vi "afslag_aan_het_kruispunt (SubVI).vi"(10 "OK Button":bool, 11 "afslag: rechtdoor: d,linksaf: l,rechtsaf: r":string) -> (3 "Boolean":bool)   [LabVIEW 2019]
uses:
  <vilib>/myRIO/Express VI/Onboard IO/PWM/PWM Express VI.xnode
  <vilib>/myRIO/Instrument Drivers/Onboard IO/PWM/vis/Set Duty Cycle and Frequency.vi
  <vilib>/myRIO/Instrument Drivers/Onboard IO/PWM/PWM.lvlib
  <vilib>/myRIO/Instrument Drivers/Onboard IO/PWM/typedefs/PWM Configuration.ctl
  <vilib>/myRIO/Common/Instrument Driver Framework/myRIO v1.0/PWM/typedefs/PWM Channels Enum.ctl
  <vilib>/myRIO/Common/Instrument Driver Framework/Utilities/typedefs/Generic FPGA Reference.ctl
  <vilib>/myRIO/Common/Instrument Driver Framework/Utilities/typedefs/myRIO v1.0 Reference.ctl
  <vilib>/myRIO/Common/Instrument Driver Framework/Utilities/typedefs/Hardware Version Enum.ctl
  <vilib>/myRIO/Common/Instrument Driver Framework/Utilities/typedefs/myRIO Generic Hardware Reference.ctl
  <vilib>/myRIO/Instrument Drivers/Onboard IO/PWM/typedefs/PWM Reference.ctl
  <vilib>/myRIO/Instrument Drivers/Onboard IO/PWM/vis/myRIO PWM Open.xnode
  <vilib>/myRIO/Common/Instrument Driver Framework/Utilities/vis/Is FPGA Ref Available.vi
  <vilib>/myRIO/Common/Instrument Driver Framework/myRIO v1.0/PWM/vis/myRIO v1.1 Open PWM.vi
  <vilib>/userDefined/High Color/nirio_resource_hc.ctl
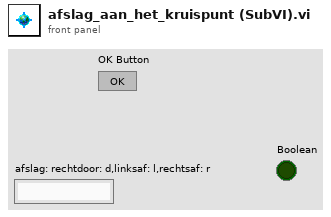
[diagram p1: front panel]
types:
  T1 = typedef "PWM.lvlib/PWM Reference.ctl" = cluster{"myRIO Reference":T2, "PWM Channels Enum":T6, "PWM Configuration":T7}
  T2 = typedef "myRIO Generic Hardware Reference.ctl" = cluster{"myRIO Model":T3, "myRIO Hardware Reference":T4}
  T3 = typedef "Hardware Version Enum.ctl" = enum16{"Unknown", "myRIO-1900", "myRIO-1950", "roboRIO", "NI ELVIS RIO CM", "ELVIS III"}
  T4 = typedef "myRIO v1.0 Reference.ctl" = cluster{"Generic FPGA Reference":T5, "Allow multiple opens":bool}
  T5 = typedef "Generic FPGA Reference.ctl" = refnum<k20>
  T6 = typedef "PWM Channels Enum.ctl" = enum16{"Not Connected", "C/PWM0", "C/PWM1", "A/PWM0", "A/PWM1", "A/PWM2", "A/PWM3", "A/PWM4", "A/PWM5", "A/PWM6", "A/PWM7", "A/PWM8", "A/PWM9", "A/PWM10", "A/PWM11", "A/PWM12", "A/PWM13", "A/PWM14", "A/PWM15", "A/PWM16", "A/PWM17", "A/PWM18", "A/PWM19", "B/PWM0", "B/PWM1", "B/PWM2", "B/PWM3", "B/PWM4", "B/PWM5", "B/PWM6", "B/PWM7", "B/PWM8", "B/PWM9", "B/PWM10", "B/PWM11", "B/PWM12", "B/PWM13", "B/PWM14", "B/PWM15", "B/PWM16", "B/PWM17", "B/PWM18", "B/PWM19", "PWM/PWM0", "PWM/PWM1", "PWM/PWM2", "PWM/PWM3", "PWM/PWM4", "PWM/PWM5", "PWM/PWM6", "PWM/PWM7", "PWM/PWM8", "PWM/PWM9"}
  T7 = typedef "PWM.lvlib/PWM Configuration.ctl" = cluster{"Frequency":dbl, "Duty Cycle":dbl}
  T8 = typedef "nirio_resource_hc.ctl" = tag
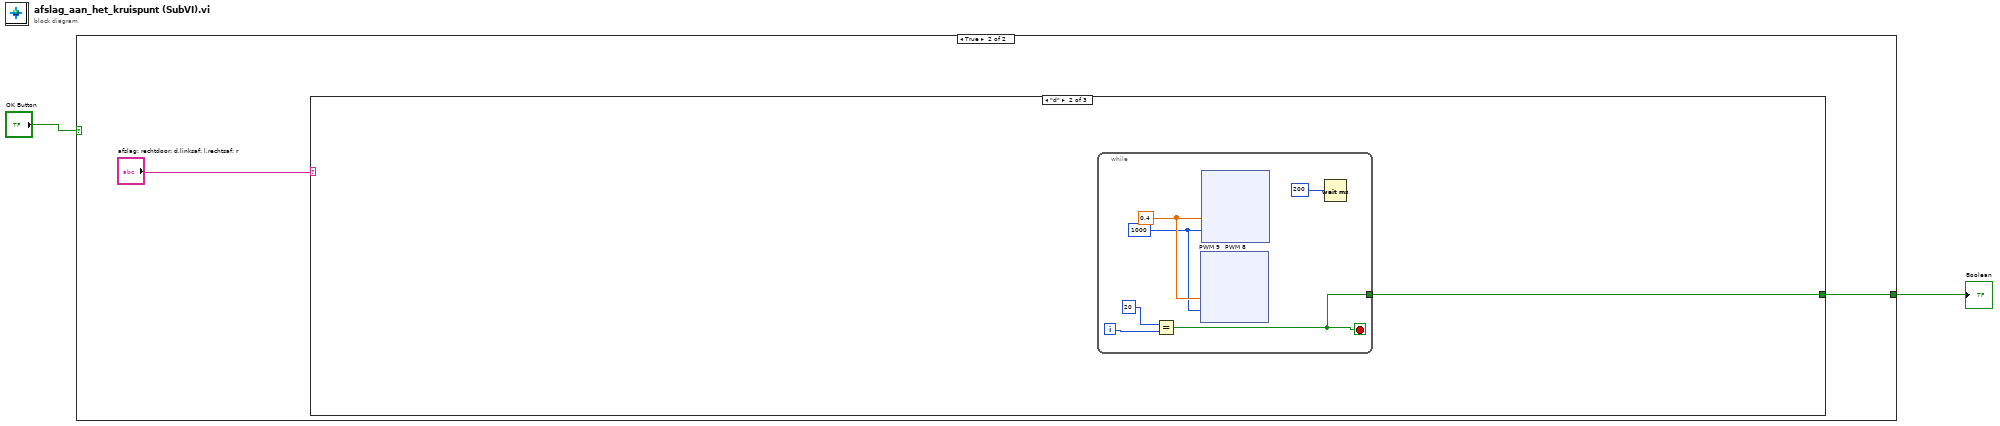
[diagram p0: block diagram]
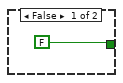
[diagram p2: hidden frame]
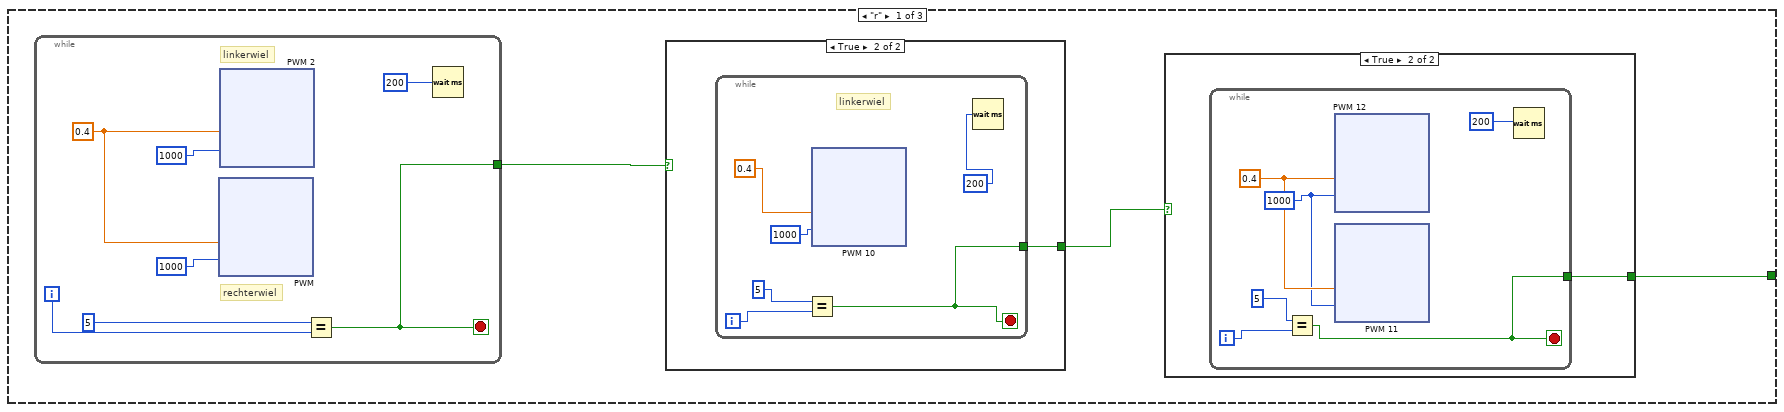
[diagram p3: hidden frame]
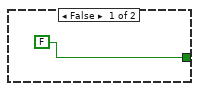
[diagram p4: hidden frame]
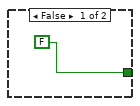
[diagram p5: hidden frame]
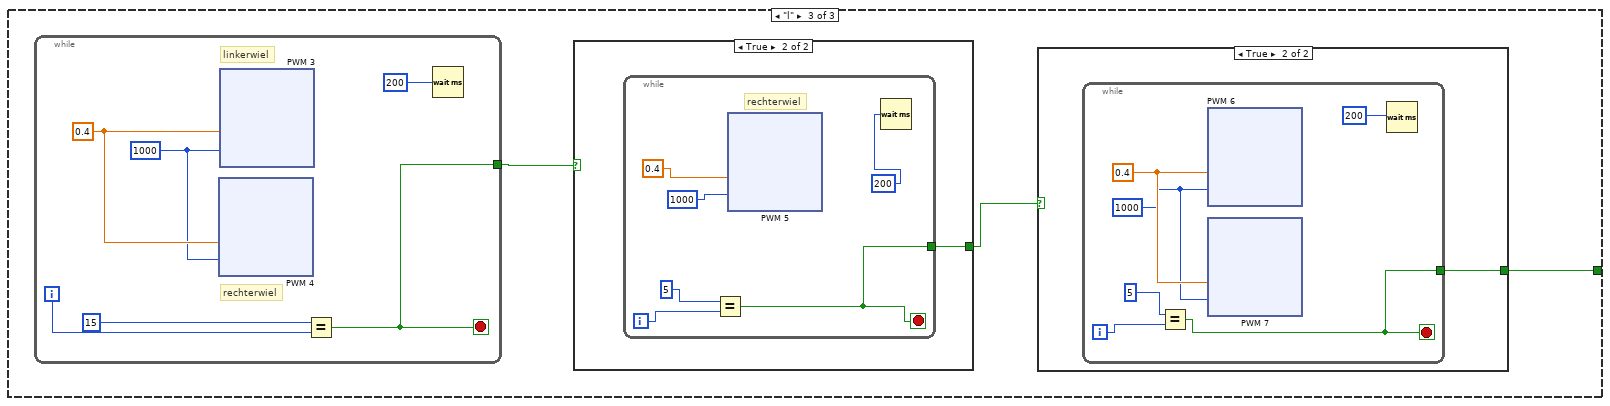
[diagram p6: hidden frame]
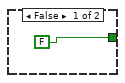
[diagram p7: hidden frame]
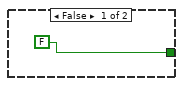
[diagram p8: hidden frame]
diagram:
  n1 = case shown="True" "OK Button" {
    tunnel: [FALSE w4] -> w1
    frame False {
    }
    frame True {
      n2 = case shown="\"d\"" "afslag: rechtdoor: d,linksaf: l,rechtsaf: r" {
        tunnel: [w6 w207 w284] -> w4
        frame "r" {
          n3 = while {
            tunnel: [w132] -> w8
            i -> [w136]
            stop <- w132 stop-if-true
            w133 = 0.4
            # "rechterwiel"
            # "linkerwiel"
            n4 = xnode "PWM"("Duty Cycle"=w133, "Frequency [Hz]"=1000) -> ()  [unwired: 1 in, 1 out]
            n5 = xnode "PWM 2"("Duty Cycle"=w133, "Frequency [Hz]"=1000) -> ()  [unwired: 1 in, 1 out]
            n6 = Equal?(x=5, y=w136) -> (x = y?=w132:bool)
            n7 = Wait (ms)(milliseconds to wait=200) -> ()  [unwired: 1 out]
          }
          n8 = case shown="True" w8 {
            tunnel: [FALSE w88] -> w7
            frame False {
            }
            frame True {
              n9 = while {
                tunnel: [w91] -> w88
                i -> [w93]
                stop <- w91 stop-if-true
                # "linkerwiel"
                n10 = Equal?(x=5, y=w93) -> (x = y?=w91:bool)
                n11 = xnode "PWM 10"("Duty Cycle"=0.4, "Frequency [Hz]"=1000) -> ()  [unwired: 1 in, 1 out]
                n12 = Wait (ms)(milliseconds to wait=200) -> ()  [unwired: 1 out]
              }
            }
          }
          n13 = case shown="True" w7 {
            tunnel: [FALSE w10] -> w6
            frame False {
            }
            frame True {
              n14 = while {
                tunnel: [w12] -> w10
                i -> [w15]
                stop <- w12 stop-if-true
                w11 = 1000
                w13 = 0.4
                n15 = Equal?(x=5, y=w15) -> (x = y?=w12:bool)
                n16 = xnode "PWM 12"("Duty Cycle"=w13, "Frequency [Hz]"=w11) -> ()  [unwired: 1 in, 1 out]
                n17 = xnode "PWM 11"("Duty Cycle"=w13, "Frequency [Hz]"=w11) -> ()  [unwired: 1 in, 1 out]
                n18 = Wait (ms)(milliseconds to wait=200) -> ()  [unwired: 1 out]
              }
            }
          }
        }
        frame "d" {
          n19 = while {
            tunnel: [w209] -> w207
            i -> [w212]
            stop <- w209 stop-if-true
            w208 = 1000
            w210 = 0.4
            n20 = Equal?(x=20, y=w212) -> (x = y?=w209:bool)
            n21 = xnode "PWM 9"("Duty Cycle"=w210, "Frequency [Hz]"=w208) -> ()  [unwired: 1 in, 1 out]
            n22 = xnode "PWM 8"("Duty Cycle"=w210, "Frequency [Hz]"=w208) -> ()  [unwired: 1 in, 1 out]
            n23 = Wait (ms)(milliseconds to wait=200) -> ()  [unwired: 1 out]
          }
        }
        frame "l" {
          n24 = while {
            tunnel: [w409] -> w286
            i -> [w413]
            stop <- w409 stop-if-true
            w408 = 1000
            w410 = 0.4
            # "rechterwiel"
            # "linkerwiel"
            n25 = xnode "PWM 4"("Duty Cycle"=w410, "Frequency [Hz]"=w408) -> ()  [unwired: 1 in, 1 out]
            n26 = xnode "PWM 3"("Duty Cycle"=w410, "Frequency [Hz]"=w408) -> ()  [unwired: 1 in, 1 out]
            n27 = Equal?(x=15, y=w413) -> (x = y?=w409:bool)
            n28 = Wait (ms)(milliseconds to wait=200) -> ()  [unwired: 1 out]
          }
          n29 = case shown="True" w286 {
            tunnel: [FALSE w366] -> w285
            frame False {
            }
            frame True {
              n30 = while {
                tunnel: [w368] -> w366
                i -> [w370]
                stop <- w368 stop-if-true
                # "rechterwiel"
                n31 = Equal?(x=5, y=w370) -> (x = y?=w368:bool)
                n32 = xnode "PWM 5"("Duty Cycle"=0.4, "Frequency [Hz]"=1000) -> ()  [unwired: 1 in, 1 out]
                n33 = Wait (ms)(milliseconds to wait=200) -> ()  [unwired: 1 out]
              }
            }
          }
          n34 = case shown="True" w285 {
            tunnel: [FALSE w288] -> w284
            frame False {
            }
            frame True {
              n35 = while {
                tunnel: [w290] -> w288
                i -> [w293]
                stop <- w290 stop-if-true
                w289 = 1000
                w291 = 0.4
                n36 = Equal?(x=5, y=w293) -> (x = y?=w290:bool)
                n37 = xnode "PWM 6"("Duty Cycle"=w291, "Frequency [Hz]"=w289) -> ()  [unwired: 1 in, 1 out]
                n38 = xnode "PWM 7"("Duty Cycle"=w291, "Frequency [Hz]"=w289) -> ()  [unwired: 1 in, 1 out]
                n39 = Wait (ms)(milliseconds to wait=200) -> ()  [unwired: 1 out]
              }
            }
          }
        }
      }
    }
  }
  "Boolean" <- w1
